vi "emi_Stop Loop w single ID err.vi"(1 "Elevated priority(F)":bool, 2 "Stop on error(T)":bool=TRUE, 5 "Loop ID in":u16, 7 "Force stop(F)":bool, 9 "error in (no error)":errorcluster) -> (6 "Loop ID out":u16, 10 "error out":errorcluster, 13 "Stop Loop":bool)   [LabVIEW 2010]
doc: "Check if loop should exit, also loggs error"
uses:
  Basic/0 - General/Error/emi_Is Error.vi
  emi_Set Status Loop.vi
  S&E reporting/emi_Send S&E Error message.vi
  emi_Read System ID.vi
  Private/_emi_GFV System ID.vi
  S&E reporting/Private/_emi_S&E Q Generator.vi
  <vilib>/Utility/error.llb/Clear Errors.vi
  Private/_emi_GFV Loop Linking.vi
  Private/_emi_GFV stop a loop so it can reset.vi
  Private/_emi_GFV Loop Enable.vi
  Private/_emi_GFV App Close.vi
  Private/_emi_GFV Loop Running.vi
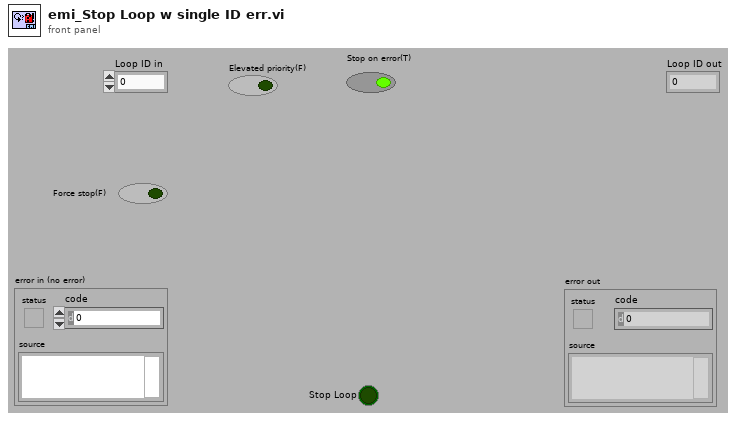
[diagram p1: front panel]
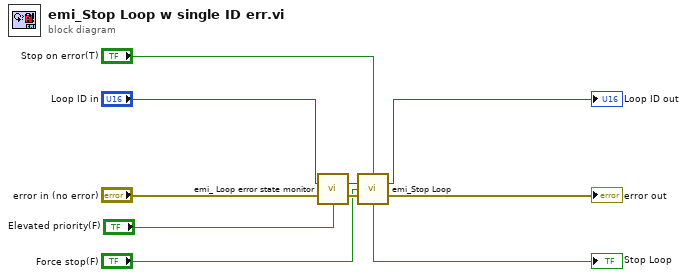
[diagram p0: block diagram]
diagram:
  n1 = call "emi_ Loop error state monitor.vi"("Loop ID in"="Loop ID in", "error in (no error)"="error in (no error)", "Elevated priority"="Elevated priority(F)") -> ("Loop ID out"=w9:u16, "error out"=w10:errorcluster)  [unwired: 11 in]
  n2 = call "emi_Stop Loop.vi"("Stop on error(T)"="Stop on error(T)", "Loop ID in"=w9, "Force stop(F)"="Force stop(F)", "error in (no error)"=w10) -> ("Loop ID out"=→"Loop ID out":u16, "error out"=→"error out":errorcluster, "Stop Loop"=→"Stop Loop":bool)  [unwired: 9 in]
